vi "Fetch Waveform Measurement (More).vi"(0 "VISA resource name":refnum<visa-resource-name>, 5 "Channel A (0:Channel 1)":u16(ring) items=["Channel 1", "Channel 2", "Channel 3", "Channel 4", "Math 1", "Math 2", "Math 3", "Math 4", "Reference 1", "Reference 2", "Reference 3", "Reference 4"], 7 "Function (0:Area)":u16(ring) items=["Area", "Burst Width", "Cyc Area", "Phase"], 9 "Channel B (1:Channel 2)":u16(ring)=1 items=["Channel 1", "Channel 2", "Channel 3", "Channel 4", "Math 1", "Math 2", "Math 3", "Math 4", "Reference 1", "Reference 2", "Reference 3", "Reference4"], 11 "error in (no error)":errorcluster) -> (4 "VISA resource name out":refnum<visa-resource-name>, 6 "Measurement":dbl, 15 "error out":errorcluster)   [LabVIEW 2015, in "Tektronix 7000 Series.lvlib"]
doc: "Initiates a waveform acquisition on the specified channels and returns a <B>Measurement</B> value. Use the Fetch Waveform Measurement VI separately for any other waveform measurement on a channel without initiating another acquisition."
uses:
  <instrlib>/Tektronix 7000 Series/Tektronix 7000 Series.lvlib
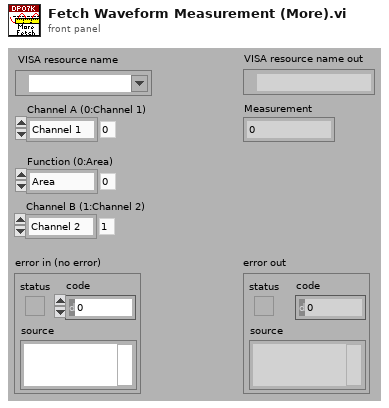
[diagram p1: front panel]
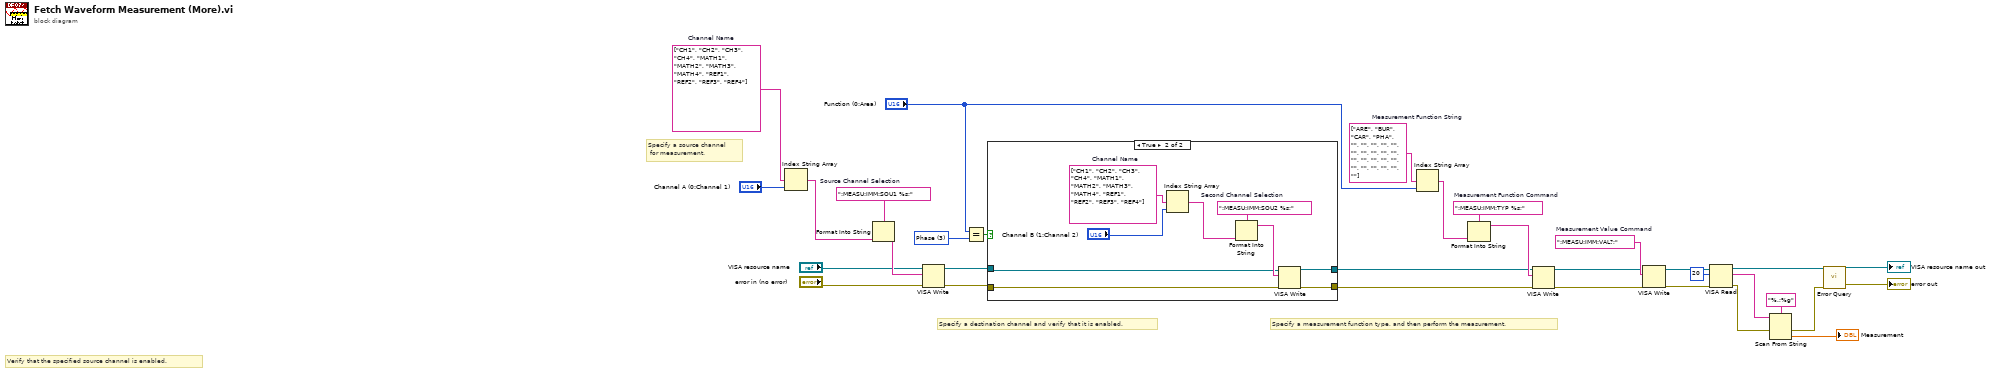
[diagram p0: block diagram]
diagram:
  w5 = u16 3 items=["Area", "Burst Width", "Cyc Area", "Phase"] ("Function(0:Amplitude)")
  w11 = string[] ["CH1", "CH2", "CH3", "CH4", "MATH1", "MATH2", "MATH3", "MATH4", "REF1", "REF2", "REF3", "REF4"]  # Channel Name
  w14 = ":MEASU:IMM:SOU1 %s;"  # Source Channel Selection
  w26 = ":MEASU:IMM:VAL?;"  # Measurement Value Command
  w31 = ":MEASU:IMM:TYP %s;"  # Measurement Function Command
  w32 = string[] ["ARE", "BUR", "CAR", "PHA", "", "", "", "", "", "", "", "", "", "", "", "", "", "", "", "", "", "", "", "", ""]  # Measurement Function String
  # "Specify a source channel\n for measurement."
  # "Specify a measurement function type, and then perform the measurement."
  # "Specify a destination channel and verify that it is enabled."
  # "Verify that the specified source channel is enabled."
  n1 = Index String Array(1:"Channel A (0:Channel 1)", 2:w11) -> (0:w15:string)  [unwired: 1 in]
  n2 = Format Into String(format string=w14, w15) -> (resulting string=w13:string)  [unwired: 2 in, 1 out]
  n3 = VISA Write(VISA resource name="VISA resource name", write buffer=w13, error in (no error)="error in (no error)") -> (VISA resource name out=w17:refnum<visa-resource-name>, error out=w16:errorcluster)  [unwired: 1 out]
  n4 = Equal?(x="Function (0:Area)", y=w5) -> (x = y?=w10:bool)
  n5 = case shown="True" w10 {
    tunnel: w17 -> [w34 w37]
    tunnel: w16 -> [w33 w36]
    tunnel: [w34 w39] -> w28
    tunnel: [w33 w38] -> w27
    frame False {
    }
    frame True {
      w40 = string[] ["CH1", "CH2", "CH3", "CH4", "MATH1", "MATH2", "MATH3", "MATH4", "REF1", "REF2", "REF3", "REF4"]  # Channel Name
      w42 = ":MEASU:IMM:SOU2 %s;"  # Second Channel Selection
      n6 = Index String Array(1:"Channel B (1:Channel 2)", 2:w40) -> (0:w43:string)  [unwired: 1 in]
      n7 = Format Into String(format string=w42, w43) -> (resulting string=w41:string)  [unwired: 2 in, 1 out]
      n8 = VISA Write(VISA resource name=w37, write buffer=w41, error in (no error)=w36) -> (VISA resource name out=w39:refnum<visa-resource-name>, error out=w38:errorcluster)  [unwired: 1 out]
    }
  }
  n9 = Index String Array(1:"Function (0:Area)", 2:w32) -> (0:w30:string)  [unwired: 1 in]
  n10 = Format Into String(format string=w31, w30) -> (resulting string=w29:string)  [unwired: 2 in, 1 out]
  n11 = VISA Write(VISA resource name=w28, write buffer=w29, error in (no error)=w27) -> (VISA resource name out=w19:refnum<visa-resource-name>, error out=w18:errorcluster)  [unwired: 1 out]
  n12 = VISA Write(VISA resource name=w19, write buffer=w26, error in (no error)=w18) -> (VISA resource name out=w25:refnum<visa-resource-name>, error out=w24:errorcluster)  [unwired: 1 out]
  n13 = VISA Read(VISA resource name=w25, byte count=u32 20, error in (no error)=w24) -> (VISA resource name out=w7:refnum<visa-resource-name>, read buffer=w22:string, error out=w4:errorcluster)  [unwired: 1 out]
  n14 = Scan From String(format string="%.;%g", input string=w22, error in=w4) -> (error out=w3:errorcluster, output 1=→"Measurement":dbl)  [unwired: 2 in, 2 out]
  n15 = call <instrlib>:"Error Query.vi"("error in (no error)"=w3, "VISA resource name"=w7) -> ("error out"=→"error out":errorcluster, "VISA resource name out"=→"VISA resource name out":refnum<visa-resource-name>)  [unwired: 6 in, 2 out]
